vi "RT Loop - System Health and Monitoring.vi"(11 "Message Queue":refnum<queue>) -> ()   [LabVIEW 2018]
uses:
  Support/Message Queue/Message Cluster.ctl
  Support/Message Queue/Message.ctl
  Controls/VTF Sensors.ctl
  Globals/Global - Configuration Options.vi
  <vilib>/nisyscfg/Close (System).vi
  <vilib>/NI_Real-Time Target Support.lvlib
  <vilib>/nisyscfg/nisyscfg.lvlib
  <resource>/objmgr/nisysapi.rc
  support/Message Queue/Message Queue.lvlib
panel:
  out "09AMBOutTemp":dbl
  out "00CylCompPres":dbl
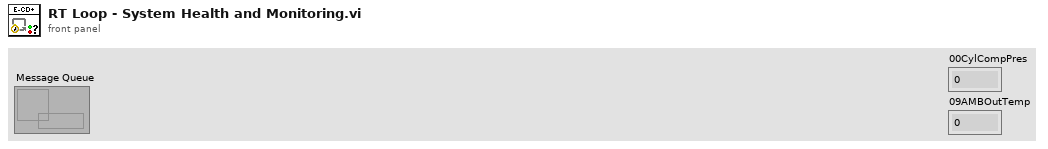
[diagram p1: front panel]
types:
  T1 = typedef "NI_Real-Time Target Support.lvlib/RT CPU Load.ctl" = cluster{"Total (%)":dbl, "Time Critical (%)":dbl, "Timed Structures (%)":dbl, "High (%)":dbl, "Above Normal (%)":dbl, "Normal (%)":dbl, "Background (%)":dbl, "Idle (%)":dbl, "ISR (%)":dbl}
  T2 = typedef "VTF Sensors.ctl" = cluster{"TJM Temp":dbl, "BrgM Temp":dbl, "Ambient Temp":dbl, "Vessel Temp":dbl}
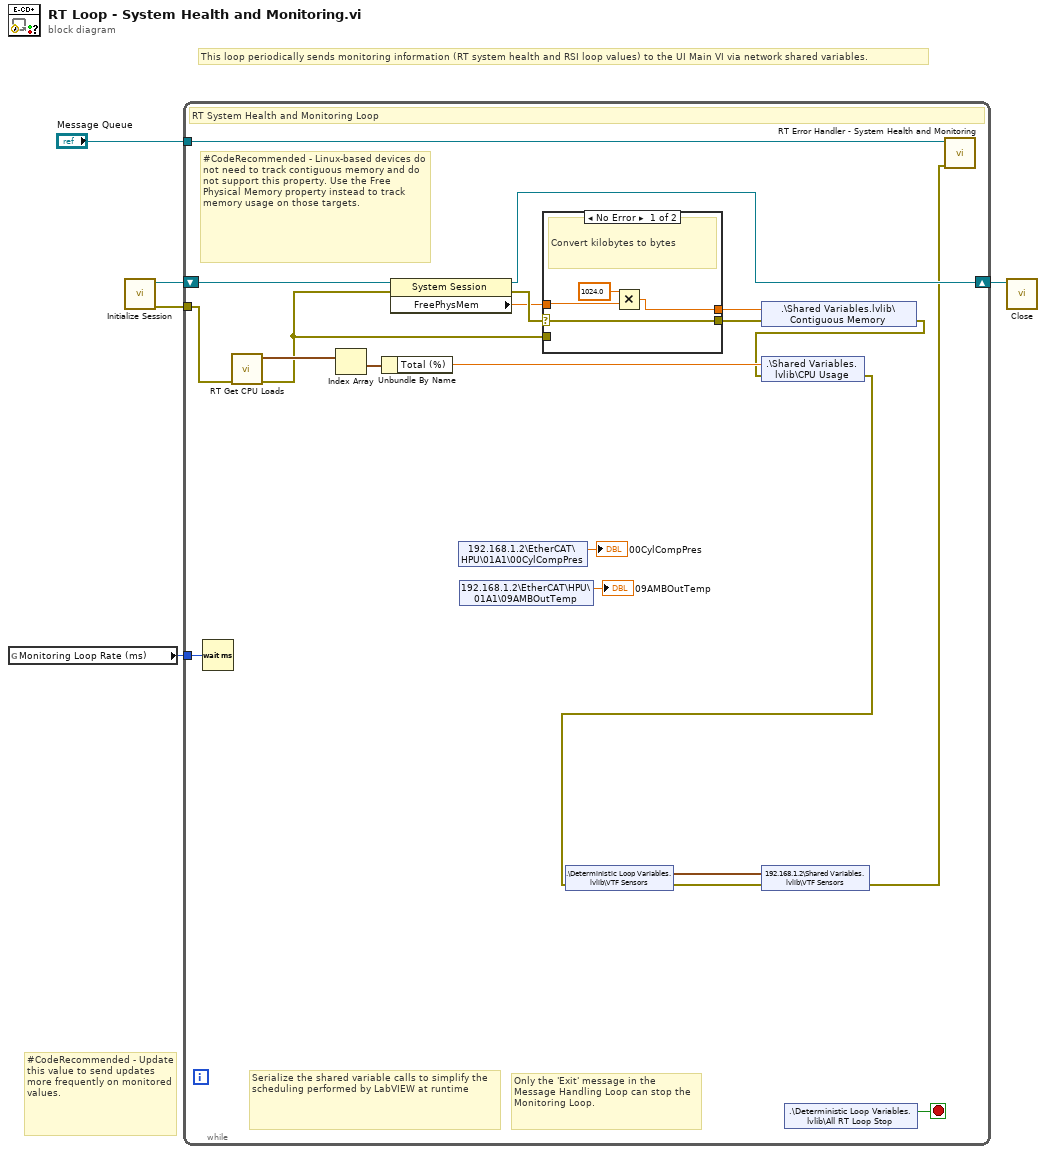
[diagram p0: block diagram]
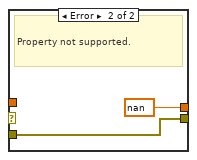
[diagram p2: hidden frame]
diagram:
  # "#CodeRecommended - Update this value to send updates more frequently on monitored values."
  # "This loop periodically sends monitoring information (RT system health and RSI loop values) to the UI Main VI via network shared variables."
  n1 = global read "Global - Configuration Options.vi" "Monitoring Loop Rate (ms)"() -> (w4:u32)
  n2 = call <vilib>:"Initialize Session.vi"() -> ("error out"=w1:errorcluster, "Session out"=w3:refnum<k21>)  [unwired: 10 in]
  n3 = while {
    tunnel: "Message Queue" -> [w23]
    tunnel: w4 -> [w22]
    shift-right: [w12] -> w2
    shift-left: w3 -> [w19]
    tunnel: w1 -> [w18]
    stop <- w21 stop-if-true
    # "#CodeRecommended - Linux-based devices do not need to track contiguous memory and do not support this property. Use the Free Physical Memory property instead to track memory usage on those targets."
    # "Serialize the shared variable calls to simplify the scheduling performed by LabVIEW at runtime"
    # "Only the 'Exit' message in the  Message Handling Loop can stop the Monitoring Loop."
    # "RT System Health and Monitoring Loop"
    n4 = Wait (ms)(milliseconds to wait=w22) -> ()  [unwired: 1 out]
    n5 = call <vilib>:"RT Get CPU Loads.vi"("error in (no error)"=w18) -> ("error out"=w15:errorcluster, "CPU loads"=w26:T1[])  [unwired: 9 in]
    n6 = Index Array(array=w26) -> (element=w25:T1)  [unwired: 1 in]
    n7 = Unbundle By Name(w25) -> ("Total (%)"=w24:dbl)
    n8 = property class="System Session"(reference=w19, error in=w15) -> (reference out=w12:refnum<k21>, error out=w17:errorcluster, "FreePhysMem"=w16:dbl)
    n9 = shared-variable "192.168.1.2\\EtherCAT\\HPU\\01A1\\00CylCompPres"() -> (→"00CylCompPres":dbl)  [unwired: 1 in, 1 out]
    n10 = shared-variable "192.168.1.2\\EtherCAT\\HPU\\01A1\\09AMBOutTemp"() -> (→"09AMBOutTemp":dbl)  [unwired: 1 in, 1 out]
    n11 = case shown="No Error" w17 {
      selector: w17 -> [w27 _]
      tunnel: w16 -> [w29 _]
      tunnel: [w28 nan] -> w14
      tunnel: [w27 w31] -> w13
      tunnel: w15 -> [_ w31]
      frame No Error {
        # "Convert kilobytes to bytes"
        n12 = Multiply(x=1024.0, y=w29) -> (x*y=w28:dbl)
      }
      frame Error {
        # "Property not supported."
      }
    }
    n13 = shared-variable ".\\Shared Variables.lvlib\\Contiguous Memory"(w14, error in=w13) -> (error out=w20:errorcluster)
    n14 = shared-variable ".\\Shared Variables.lvlib\\CPU Usage"(w24, error in=w20) -> (error out=w10:errorcluster)
    n15 = shared-variable ".\\Deterministic Loop Variables.lvlib\\VTF Sensors"(error in=w10) -> (w8:T2, error out=w9:errorcluster)
    n16 = shared-variable "192.168.1.2\\Shared Variables.lvlib\\VTF Sensors"(w8, error in=w9) -> (error out=w11:errorcluster)
    n17 = shared-variable ".\\Deterministic Loop Variables.lvlib\\All RT Loop Stop"() -> (w21:bool)  [unwired: 1 in, 1 out]
    n18 = call "RT Error Handler - System Health and Monitoring.vi"("error in (no error)"=w11, "Message Queue"=w23) -> ()  [unwired: 9 in, 1 out]
  }
  n19 = call-poly <vilib>:"Close.vi"("Session in"=w2) -> ()  [unwired: 10 in, 1 out]
